vi "Define Equation.vi"(5 "target RHS":refnum<class "NI_RHS.lvclass">, 7 "target PDE":refnum<class "NI_PDE.lvclass">, 8 "error in (no error)":errorcluster, 9 "RHS":variant, 10 "parameter":variant, 11 "PDE in":refnum<class "NI_PDE.lvclass">) -> (0 "error out":errorcluster, 3 "PDE out":refnum<class "NI_PDE.lvclass">)   [LabVIEW 2017, in "NI_PDE.lvlib" / "NI_PDE.lvclass"]
uses:
  <vilib>/gmath/pde.llb/PDEClass/NI_PDE.lvclass
  <vilib>/gmath/pde.llb/RHSClass/NI_RHS.lvclass
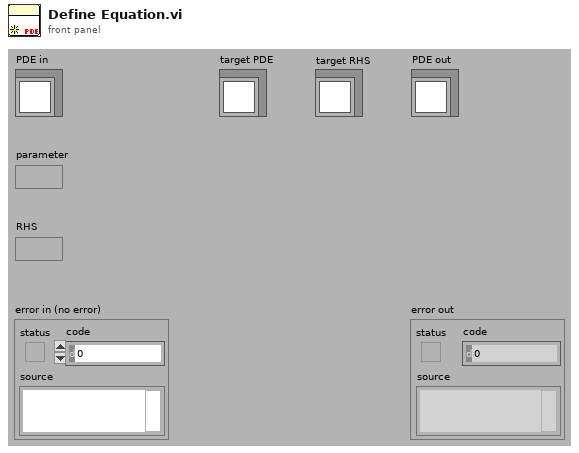
[diagram p1: front panel]
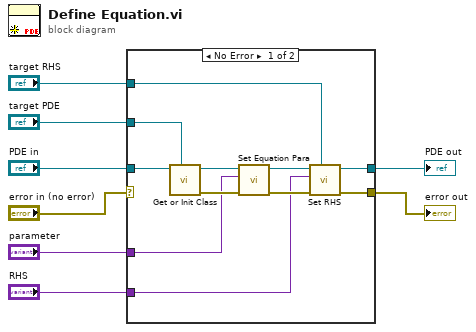
[diagram p0: block diagram]
diagram:
  n1 = case shown="No Error" "error in (no error)" {
    selector: "error in (no error)" -> [_ w21]
    tunnel: "PDE in" -> [w13 w20]
    tunnel: [w15 w20] -> w8
    tunnel: [w14 w21] -> w7
    tunnel: "target RHS" -> [w9 _]
    tunnel: "RHS" -> [w11 _]
    tunnel: "target PDE" -> [w10 _]
    tunnel: "parameter" -> [w12 _]
    frame No Error {
      n2 = call <vilib>:"Get or Init Class.vi"("target PDE"=w10, "PDE in"=w13) -> ("error out"=w19:errorcluster, "PDE out"=w18:refnum<class "NI_PDE.lvclass">)  [unwired: 2 in, 6 out]
      n3 = call-dynamic "Set Equation Para.vi"("error in (no error)"=w19, "parameter"=w12, "PDE in"=w18) -> ("error out"=w17:errorcluster, "PDE out"=w16:refnum<class "NI_PDE.lvclass">)  [unwired: 7 out]
      n4 = call <vilib>:"Set RHS.vi"("target RHS"=w9, "error in (no error)"=w17, "RHS"=w11, "PDE in"=w16) -> ("error out"=w14:errorcluster, "PDE out"=w15:refnum<class "NI_PDE.lvclass">)  [unwired: 6 out]
    }
    frame Error {
    }
  }
  "PDE out" <- w8
  "error out" <- w7
